vi "Read Comma Separated String.vi"(7 "key":string, 8 "error in (no error)":errorcluster, 9 "default value":string, 11 "Configuration File In":refnum<class "Configuration File.lvclass">) -> (0 "error out":errorcluster, 1 "values":string[](array[string]), 3 "Configuration File Out":refnum<class "Configuration File.lvclass">)   [LabVIEW 2020, in "Configuration File.lvclass"]
doc: "High-level function for reading configuration file data from process class. If the specified key is not present, it is added with the configured default value."
uses:
  Configuration File.lvclass
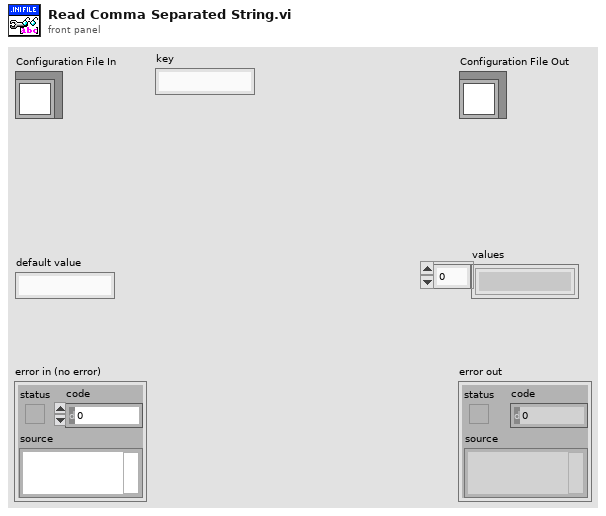
[diagram p1: front panel]
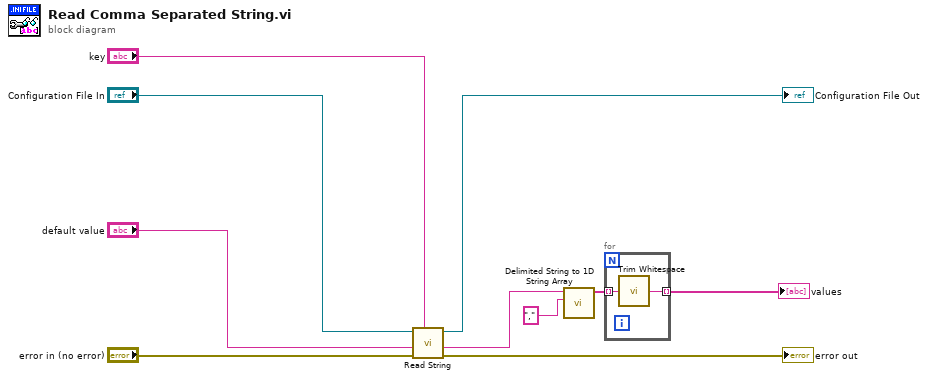
[diagram p0: block diagram]
diagram:
  n1 = call-dynamic "Read String.vi"("key"="key", "error in (no error)"="error in (no error)", "default value"="default value", "Configuration File In"="Configuration File In") -> ("error out"=→"error out":errorcluster, "value"=w4:string, "Configuration File Out"=→"Configuration File Out":refnum<class "Configuration File.lvclass">)  [unwired: 5 in]
  n2 = call <vilib>:"Delimited String to 1D String Array.vi"("delimiter"=",", "delimited string"=w4) -> ("string array"=w2:string[])  [unwired: 9 in]
  n3 = for {
    tunnel: w2 -> [w12] mode=indexing
    tunnel: [w11] -> w1 mode=indexing
    n4 = call <vilib>:"Trim Whitespace.vi"("string"=w12) -> ("trimmed string"=w11:string)  [unwired: 1 in]
  }
  "values" <- w1
